vi "Shutter Messenger.vi"(0 "Notifier Name":string, 2 "Quick Status":bool, 11 "Action":T1) -> (4 "Notifier Name Dup":string, 8 "Shutter Status":T1)   [LabVIEW 2016]
uses:
  Shutter Controls/Shutter Actions.ctl
  Shutter Controls/Shutter Notifier Element.ctl
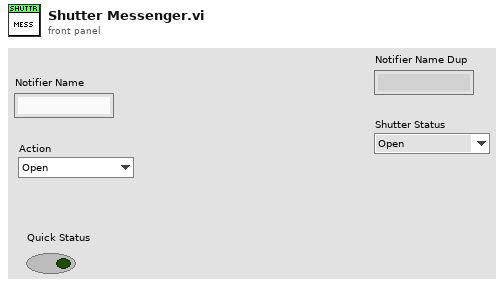
[diagram p1: front panel]
types:
  T1 = typedef "Shutter Actions.ctl" = enum16{"Open", "Close", "Toggle", "Status", "Quit"}
  T2 = typedef "Shutter Notifier Element.ctl" = cluster{"Action":T1, "Status":T1, "Received?":bool}
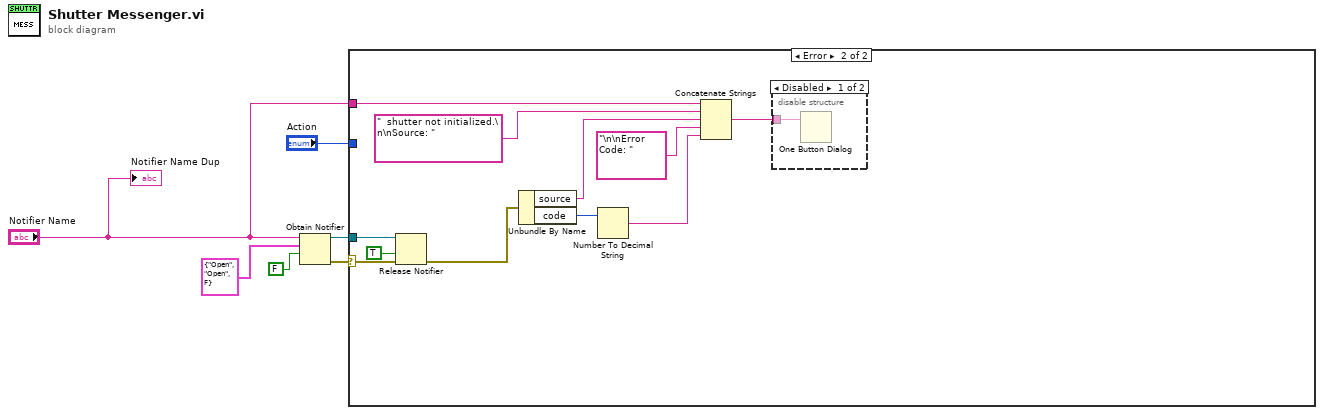
[diagram p0: block diagram]
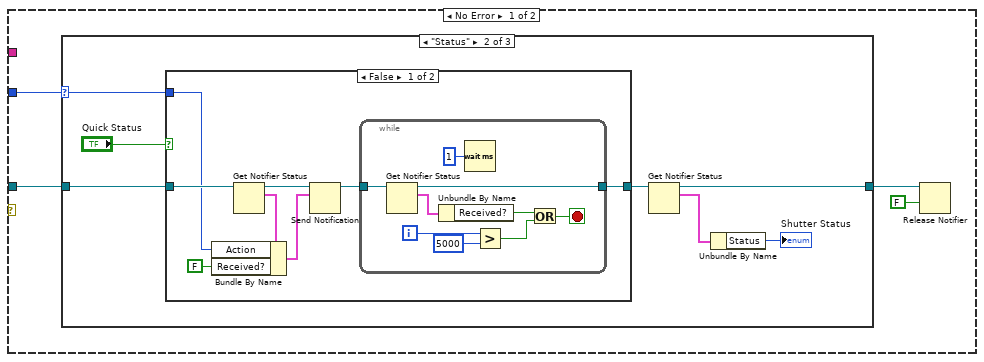
[diagram p2: hidden frame]
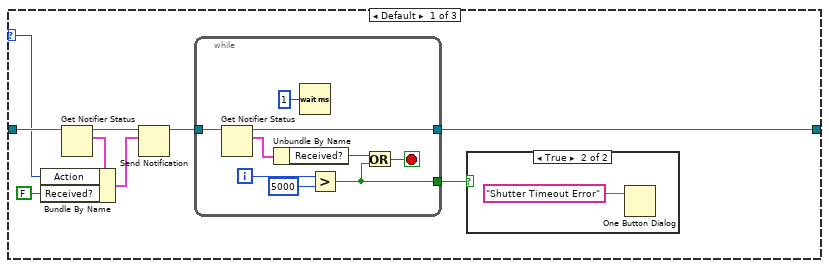
[diagram p3: hidden frame]
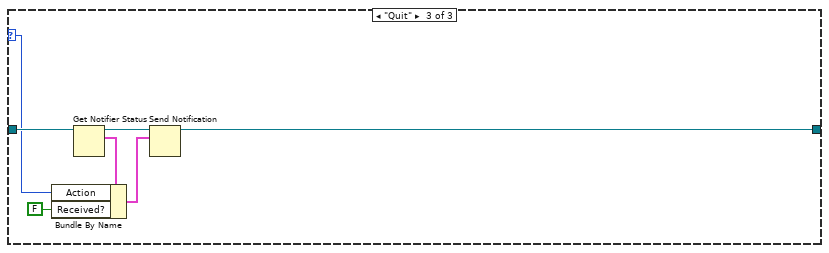
[diagram p6: hidden frame]
diagram:
  n1 = Obtain Notifier(name (unnamed)="Notifier Name", notification data type=T2 {"Action"=enum."Open", "Status"=enum."Open", "Received?"=FALSE} ("Shutter Notifier Element"), create if not found? (T)=FALSE) -> (notifier out=w6:refnum<notifier>, error out=w3:errorcluster)  [unwired: 1 in, 1 out]
  n2 = case shown="Error" w3 {
    selector: w3 -> [_ w68]
    tunnel: w6 -> [w10 w72]
    tunnel: "Action" -> [w9 _]
    tunnel: "Notifier Name" -> [_ w63]
    frame No Error {
      n3 = case shown="\"Status\"" w9 {
        selector: w9 -> [w11 w33 w56]
        tunnel: w10 -> [w19 w36 w57]
        tunnel: [w12 w34 w55] -> w8
        frame Default {
          n4 = Get Notifier Status(notifier=w19) -> (notifier out=w16:refnum<notifier>, current notification=w18:T2)  [unwired: 1 in, 3 out]
          n5 = Bundle By Name(cluster=w18, "Action"=w11, "Received?"=FALSE) -> (w15:T2)
          n6 = Send Notification(notification=w15, notifier=w16) -> (notifier out=w14:refnum<notifier>)  [unwired: 1 in, 1 out]
          n7 = while {
            tunnel: w14 -> [w29]
            tunnel: [w27] -> w12
            tunnel: [w21] -> w13
            i -> [w24]
            stop <- w22 stop-if-true
            n8 = Get Notifier Status(notifier=w29) -> (notifier out=w27:refnum<notifier>, current notification=w28:T2)  [unwired: 1 in, 3 out]
            n9 = Unbundle By Name(w28) -> ("Received?"=w25:bool)
            n10 = Wait (ms)(milliseconds to wait=u32 1) -> ()  [unwired: 1 out]
            n11 = Greater?(x=w24, y=5000) -> (0:w21:bool)
            n12 = Or(x=w25, y=w21) -> (x .or. y?=w22:bool)
          }
          n13 = case shown="True" w13 {
            frame False {
            }
            frame True {
              n14 = One Button Dialog(message="Shutter Timeout Error" ("string")) -> ()  [unwired: 1 in, 1 out]
            }
          }
        }
        frame "Status" {
          n15 = case shown="False" "Quick Status" {
            tunnel: w36 -> [w44 w54]
            tunnel: [w38 w54] -> w35
            tunnel: w33 -> [w37 _]
            frame False {
              n16 = Get Notifier Status(notifier=w44) -> (notifier out=w41:refnum<notifier>, current notification=w43:T2)  [unwired: 1 in, 3 out]
              n17 = Bundle By Name(cluster=w43, "Action"=w37, "Received?"=FALSE) -> (w40:T2)
              n18 = Send Notification(notification=w40, notifier=w41) -> (notifier out=w39:refnum<notifier>)  [unwired: 1 in, 1 out]
              n19 = while {
                tunnel: w39 -> [w53]
                tunnel: [w51] -> w38
                i -> [w48]
                stop <- w46 stop-if-true
                n20 = Get Notifier Status(notifier=w53) -> (notifier out=w51:refnum<notifier>, current notification=w52:T2)  [unwired: 1 in, 3 out]
                n21 = Unbundle By Name(w52) -> ("Received?"=w49:bool)
                n22 = Wait (ms)(milliseconds to wait=u32 1) -> ()  [unwired: 1 out]
                n23 = Greater?(x=w48, y=5000) -> (0:w45:bool)
                n24 = Or(x=w49, y=w45) -> (x .or. y?=w46:bool)
              }
            }
            frame True {
            }
          }
          n25 = Get Notifier Status(notifier=w35) -> (notifier out=w34:refnum<notifier>, current notification=w32:T2)  [unwired: 1 in, 3 out]
          n26 = Unbundle By Name(w32) -> ("Status"=→"Shutter Status":T1)
        }
        frame "Quit" {
          n27 = Get Notifier Status(notifier=w57) -> (notifier out=w60:refnum<notifier>, current notification=w61:T2)  [unwired: 1 in, 3 out]
          n28 = Bundle By Name(cluster=w61, "Action"=w56, "Received?"=FALSE) -> (w59:T2)
          n29 = Send Notification(notification=w59, notifier=w60) -> (notifier out=w55:refnum<notifier>)  [unwired: 1 in, 1 out]
        }
      }
      n30 = Release Notifier(notifier=w8, force destroy? (F)=FALSE) -> ()  [unwired: 1 in, 3 out]
    }
    frame Error {
      n31 = Release Notifier(notifier=w72, force destroy? (F)=TRUE, error in (no error)=w68) -> (error out=w62:errorcluster)  [unwired: 2 out]
      n32 = Unbundle By Name(w62) -> ("source"=w67:string, "code"=w66:i32)
      n33 = Number To Decimal String(number=w66) -> (decimal integer string=w64:string)  [unwired: 1 in]
      n34 = Concatenate Strings(w63, "  shutter not initialized.\n\nSource: " ("message"), w67, "\n\nError Code: " ("message"), w64) -> (w69:string)
      n35 = disable-structure shown="Disabled" {
        disable-tunnel: w69 -> [w73 _]
        frame Disabled {
          n36 = One Button Dialog(message=w73) -> ()  [unwired: 1 in, 1 out]
        }
        frame Enabled {
        }
      }
    }
  }
  "Notifier Name Dup" <- "Notifier Name"
